vi "name data.vi"(8 "error in (no error)":errorcluster, 11 "Dynamic Data":dynamicdata(waveform)) -> (0 "error out":errorcluster, 3 "Output":dynamicdata(waveform))   [LabVIEW 2011]
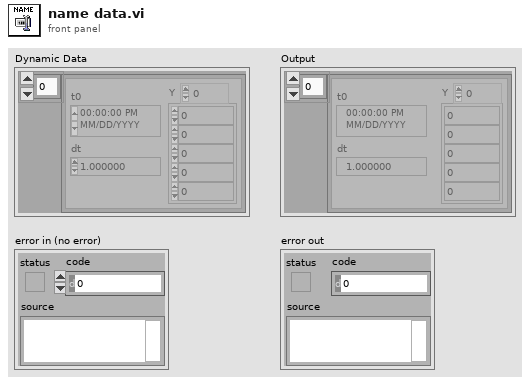
[diagram p1: front panel]
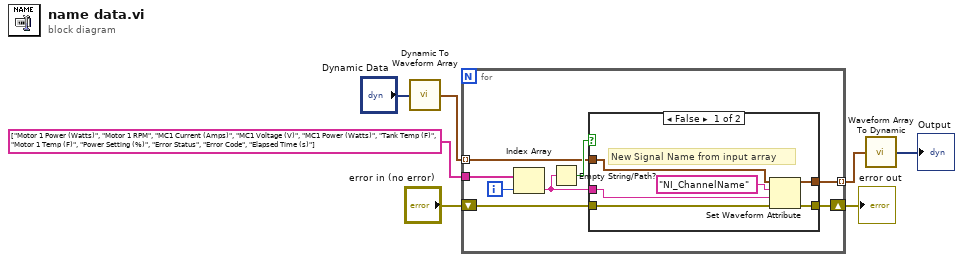
[diagram p0: block diagram]
diagram:
  n1 = call <vilib>:"Dynamic To Waveform Array.vi"("Input"="Dynamic Data") -> ("Output"=w1:waveform(dbl)[])  [unwired: 4 in]
  n2 = for {
    tunnel: w1 -> [w12] mode=indexing
    tunnel: string[] ["Motor 1 Power (Watts)", "Motor 1 RPM", "MC1 Current (Amps)", "MC1 Voltage (V)", "MC1 Power (Watts)", "Tank Temp (F)", "Motor 1 Temp (F)", "Power Setting (%)", "Error Status", "Error Code", "Elapsed Time (s)"] ("New Signal Names") -> [w15]
    shift-right: [w9] -> w6
    shift-left: "error in (no error)" -> [w11]
    tunnel: [w8] -> w2 mode=indexing
    i -> [w14]
    n3 = Index Array(array=w15, index=w14) -> (element=w10:string)
    n4 = Empty String/Path?(string/path=w10) -> (empty?=w13:bool)
    n5 = case shown="False" w13 {
      tunnel: w12 -> [w21 w23]
      tunnel: w11 -> [w20 w22]
      tunnel: [w17 w22] -> w9
      tunnel: [w18 w23] -> w8
      tunnel: w10 -> [w19 _]
      frame False {
        # "New Signal Name from input array"
        n6 = Set Waveform Attribute(4:w20, 5:w19, 6:"NI_ChannelName", 7:w21) -> (0:w17:errorcluster, 3:w18:waveform(dbl))  [unwired: 1 out]
      }
      frame True {
        # "No Signal Name in input array.\nUse original Signal Name."
      }
    }
  }
  "error out" <- w6
  n7 = call <vilib>:"Waveform Array To Dynamic.vi"("Input"=w2) -> ("Output"=→"Output":dynamicdata)  [unwired: 4 in]
